vi "Send Data Notification.vi"(7 "Notifier in":refnum<notifier>, 9 "Low Limit":dbl, 10 "High Limit":dbl, 11 "temperature":dbl) -> (0 "error out":errorcluster)   [LabVIEW 2023]
doc: "Bundles the data and sends the notification for the display."
uses:
  controls/Simulated Data.ctl
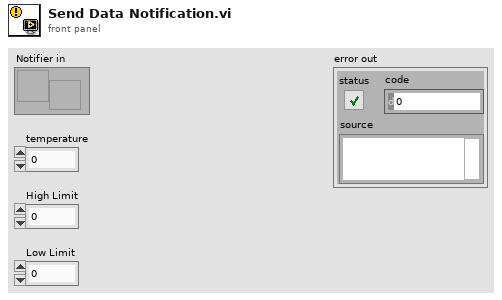
[diagram p1: front panel]
types:
  T1 = typedef "Simulated Data.ctl" = cluster{"temperature":dbl, "High Limit":dbl, "Low Limit":dbl}
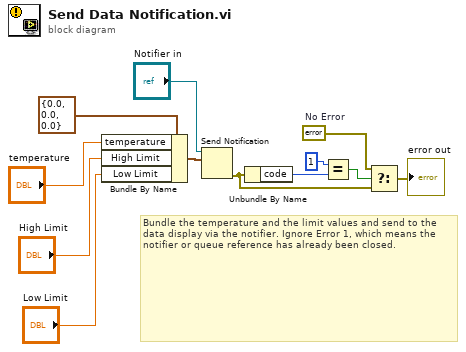
[diagram p0: block diagram]
diagram:
  w5 = errorcluster {"status"=FALSE, "code"=0, "source"=""}  # No Error
  # "Bundle the temperature and the limit values and send to the data display via the notifier. Ignore Error 1, which means the notifier or queue reference has already been closed."
  n1 = Bundle By Name(cluster=T1 {"temperature"=0.0, "High Limit"=0.0, "Low Limit"=0.0} ("output cluster"), "temperature"="temperature", "High Limit"="High Limit", "Low Limit"="Low Limit") -> (w11:T1)
  n2 = Send Notification(notification=w11, notifier="Notifier in") -> (error out=w4:errorcluster)  [unwired: 1 in, 1 out]
  n3 = Unbundle By Name(w4) -> ("code"=w1:i32)
  n4 = Equal?(x=1, y=w1) -> (x = y?=w3:bool)
  n5 = Select(t=w5, s=w3, f=w4) -> (s? t:f=→"error out":errorcluster)
